vi "FL_Zones_Loc_Get_n_Norm.vi"(8 "Amount of active segments":u32, 9 "Zones presence array in":bool[](array[boolean]), 10 "Zones allocation array in":i32[](array[numeric]), 11 "Current segment' number":u32) -> (0 "Zones normalized allocation cluster out":T1, 1 "Zones presence array out":bool[](array[boolean]), 2 "Zones allocation array out":i32[](array[numeric]), 3 "Zones presence indicator cluster out":T2, 4 "Zones normalized allocation array out":dbl[](array[numeric]))   [LabVIEW 2016]
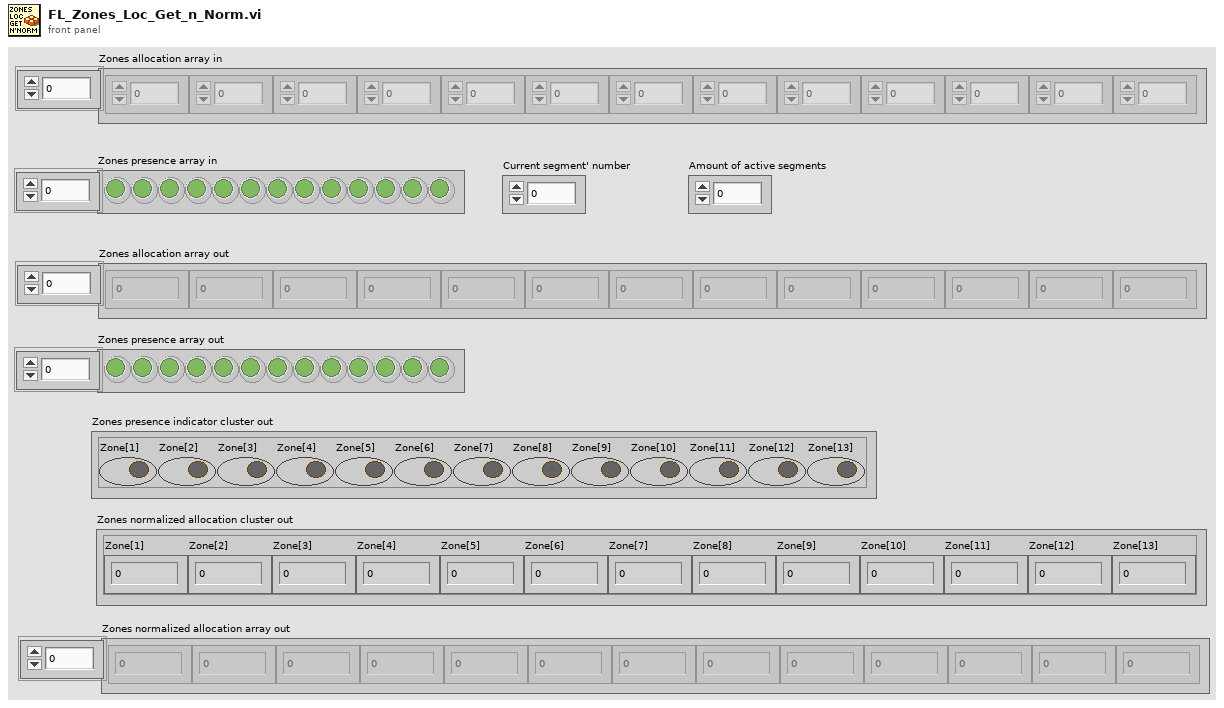
[diagram p1: front panel]
types:
  T1 = cluster{"Zone[1]":dbl, "Zone[2]":dbl, "Zone[3]":dbl, "Zone[4]":dbl, "Zone[5]":dbl, "Zone[6]":dbl, "Zone[7]":dbl, "Zone[8]":dbl, "Zone[9]":dbl, "Zone[10]":dbl, "Zone[11]":dbl, "Zone[12]":dbl, "Zone[13]":dbl}
  T2 = cluster{"Zone[1]":bool, "Zone[2]":bool, "Zone[3]":bool, "Zone[4]":bool, "Zone[5]":bool, "Zone[6]":bool, "Zone[7]":bool, "Zone[8]":bool, "Zone[9]":bool, "Zone[10]":bool, "Zone[11]":bool, "Zone[12]":bool, "Zone[13]":bool}
  T3 = cluster{"Zones presence array in[0]":bool, "Zones presence array in[1]":bool, "Zones presence array in[2]":bool, "Zones presence array in[3]":bool, "Zones presence array in[4]":bool, "Zones presence array in[5]":bool, "Zones presence array in[6]":bool, "Zones presence array in[7]":bool, "Zones presence array in[8]":bool, "Zones presence array in[9]":bool, "Zones presence array in[10]":bool, "Zones presence array in[11]":bool, "Zones presence array in[12]":bool}
  T4 = cluster{"[0]":dbl, "[1]":dbl, "[2]":dbl, "[3]":dbl, "[4]":dbl, "[5]":dbl, "[6]":dbl, "[7]":dbl, "[8]":dbl, "[9]":dbl, "[10]":dbl, "[11]":dbl, "[12]":dbl}
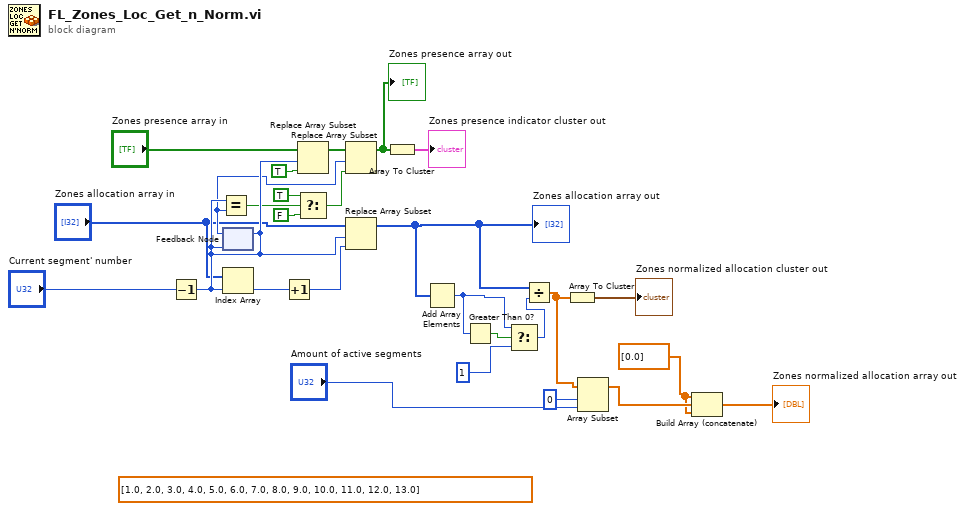
[diagram p0: block diagram]
diagram:
  w1 = dbl[] [0.0] ("element")
  (unwired) dbl[] [1.0, 2.0, 3.0, 4.0, 5.0, 6.0, 7.0, 8.0, 9.0, 10.0, 11.0, 12.0, 13.0]
  n1 = Decrement(x="Current segment' number") -> (x-1=w24:u32)
  n2 = feedback #1(w24) -> (w18:u32)
  n3 = Equal?(x=w24, y=w18) -> (x = y?=w19:bool)
  n4 = feedback-in #1(w24) -> ()
  n5 = Index Array(array="Zones allocation array in", index=w24) -> (element=w25:i32)
  n6 = Increment(x=w25) -> (x+1=w26:i32)
  n7 = Replace Array Subset(array="Zones presence array in", new element=TRUE ("new element/subarray"), index=w24) -> (w17:bool[])
  n8 = Select(t=TRUE, s=w19, f=FALSE) -> (s? t:f=w20:bool)
  n9 = Replace Array Subset(array=w17, new element=w20, index=w18) -> (w14:bool[])
  "Zones presence array out" <- w14
  n10 = Replace Array Subset(array="Zones allocation array in", new element=w26, index=w24) -> (w12:i32[])
  "Zones allocation array out" <- w12
  n11 = Array To Cluster(array=w14) -> (cluster=→"Zones presence indicator cluster out":T3)
  n12 = Add Array Elements(numeric array=w12) -> (sum=w10:i32)
  n13 = Greater Than 0?(x=w10) -> (x > 0?=w11:bool)
  n14 = Select(t=w10, s=w11, f=1) -> (s? t:f=w9:i32)
  n15 = Divide(x=w12, y=w9) -> (x/y=w6:dbl[])
  n16 = Array To Cluster(array=w6) -> (cluster=→"Zones normalized allocation cluster out":T4)
  n17 = Array Subset(array=w6, index=0, length="Amount of active segments") -> (w5:dbl[])
  n18 = Build Array (concatenate)(w1, w5, w1) -> (→"Zones normalized allocation array out":dbl[])
